vi "Prober_ChuckUpDown.vi"(8 "error in (no error)":errorcluster, 10 "Direction":enum16{"up", "down"}(ring), 11 "AlessiRel6100 in":refnum<class "AlessiRel6100.lvclass">) -> (0 "error out":errorcluster, 2 "Chuck at CONTACT?":bool=TRUE, 3 "AlessiRel6100 out":refnum<class "AlessiRel6100.lvclass">)   [LabVIEW 2018, in "AlessiRel6100.lvclass"]
uses:
  AlessiRel6100.lvclass
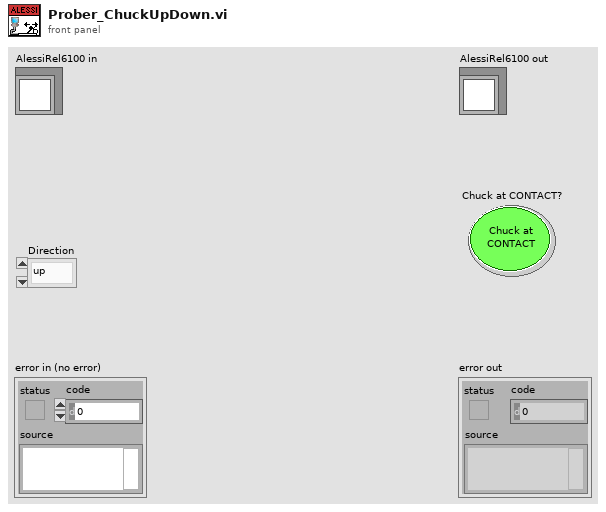
[diagram p1: front panel]
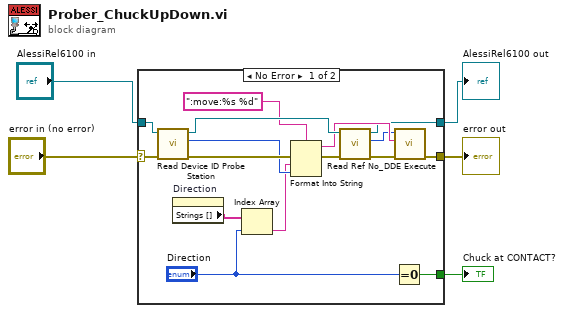
[diagram p0: block diagram]
diagram:
  n1 = case shown="No Error" "error in (no error)" {
    selector: "error in (no error)" -> [w15 w23]
    tunnel: [w11 w23] -> w3
    tunnel: "AlessiRel6100 in" -> [w10 w22]
    tunnel: [w9 _] -> w1
    tunnel: [w8 w22] -> w2
    frame No Error {
      n2 = call-dynamic "Read Device ID Probe Station.vi"("error in (no error)"=w15, "AlessiRel6100 in"=w10) -> ("error out"=w19:errorcluster, "Device ID Probe Station"=w17:u32, "AlessiRel6100 out"=w21:refnum<class "AlessiRel6100.lvclass">)  [unwired: 7 in]
      n3 = property on="Direction" class="Enum (strict)"() -> ("Strings []"=w6:string[])  [unwired: 2 in, 2 out]
      n4 = Index Array(array=w6, index="Direction") -> (element=w16:string)
      n5 = Format Into String(format string=":move:%s %d", error in=w19, w16, w17) -> (resulting string=w14:string, error out=w20:errorcluster)  [unwired: 1 in]
      n6 = call-dynamic "Read Ref No_.vi"("error in (no error)"=w20, "AlessiRel6100 in"=w21) -> ("error out"=w12:errorcluster, "Ref No."=w13:u32, "AlessiRel6100 out"=w8:refnum<class "AlessiRel6100.lvclass">)  [unwired: 7 in]
      n7 = Equal To 0?(x="Direction") -> (x = 0?=w9:bool)
      n8 = call "DDE Execute.vi"("error in (no error)"=w12, "command"=w14, "conversation refnum in"=w13) -> ("error out"=w11:errorcluster)  [unwired: 5 in, 1 out]
    }
    frame Error {
    }
  }
  "error out" <- w3
  "Chuck at CONTACT?" <- w1
  "AlessiRel6100 out" <- w2
